vi "Bytes to MiBs.vi"(1 "Numeric in":i32) -> (0 "Numeric out":dbl)   [LabVIEW 2023]
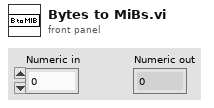
[diagram p1: front panel]
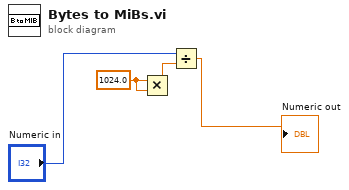
[diagram p0: block diagram]
diagram:
  w2 = 1024.0 ("x")
  n1 = Multiply(x=w2, y=w2) -> (x*y=w3:dbl)
  n2 = Divide(x="Numeric in", y=w3) -> (x/y=→"Numeric out":dbl)
